vi "Put Back Scanners.vi"(8 "error in (no error)":errorcluster, 9 "Scanner 2 in":refnum<class "Scanner.lvclass">, 10 "Scanner 1 in":refnum<class "Scanner.lvclass">, 11 "Double Scanner in":refnum<class "Double Scanner.lvclass">) -> (0 "error out":errorcluster, 3 "Double Scanner out":refnum<class "Double Scanner.lvclass">)   [LabVIEW 2017, in "Double Scanner.lvclass"]
uses:
  Double Scanner.lvclass
  Scanner/Scanner.lvclass
  Double Scanner.lvclass/Double Scanner.ctl
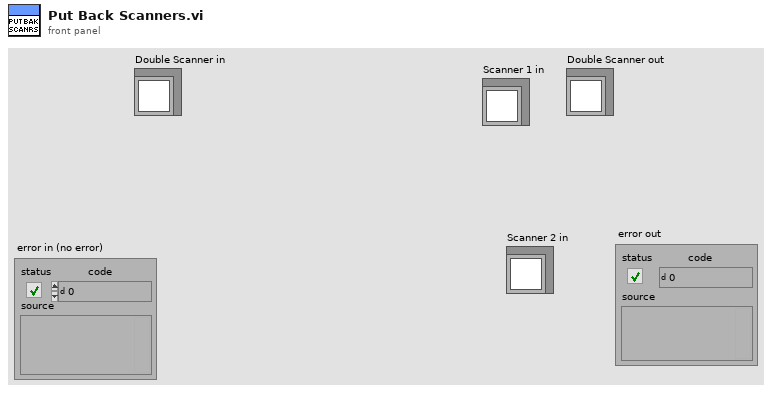
[diagram p1: front panel]
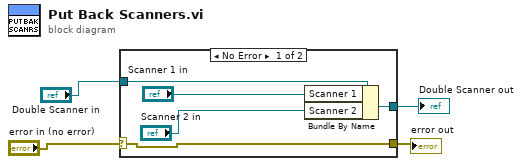
[diagram p0: block diagram]
diagram:
  n1 = case shown="No Error" "error in (no error)" {
    selector: "error in (no error)" -> [w5 w11]
    tunnel: [w7 w10] -> w4
    tunnel: "Double Scanner in" -> [w6 w10]
    tunnel: [w5 w11] -> w1
    frame No Error {
      n2 = Bundle By Name(cluster=w6, "Scanner 1"="Scanner 1 in", "Scanner 2"="Scanner 2 in") -> (w7:refnum<class "Double Scanner.lvclass">)
    }
    frame Error {
    }
  }
  "Double Scanner out" <- w4
  "error out" <- w1
